vi "RichToFlatrouteguide_Rectangle.vi"(5 "OutputClusterType":T1, 11 "InputCluster":T3) -> (3 "OutputCluster":T1)   [LabVIEW 2019, in "Generated_server.lvlib"]
uses:
  Generated_server.lvlib
  routeguide_Rectangle.ctl
  routeguide_Point.ctl
  routeguide_Rectangle_Flat.ctl
  routeguide_Point_Flat.ctl
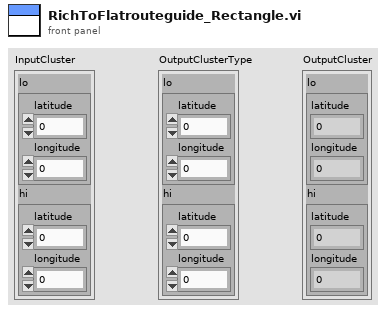
[diagram p1: front panel]
types:
  T1 = typedef "Generated_server.lvlib/routeguide_Rectangle_Flat.ctl" = cluster{"lo":T2, "hi":T2}
  T2 = typedef "Generated_server.lvlib/routeguide_Point_Flat.ctl" = cluster{"latitude":i32, "longitude":i32}
  T3 = typedef "Generated_server.lvlib/routeguide_Rectangle.ctl" = cluster{"lo":T4, "hi":T4}
  T4 = typedef "Generated_server.lvlib/routeguide_Point.ctl" = cluster{"latitude":i32, "longitude":i32}
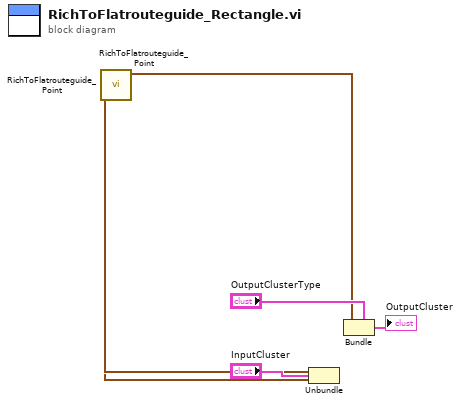
[diagram p0: block diagram]
diagram:
  n1 = Unbundle "Unbundle"("InputCluster") -> ("lo"=w4:T4, "hi"=w2:T4)
  n2 = call "RichToFlatrouteguide_Point.vi"("InputCluster"=w2) -> ("OutputCluster"=w1:T2)  [unwired: 10 in]
  n3 = call "RichToFlatrouteguide_Point.vi"("InputCluster"=w4) -> ("OutputCluster"=w3:T2)  [unwired: 10 in]
  n4 = Bundle "Bundle"(cluster="OutputClusterType", "lo"=w3, "hi"=w1) -> (→"OutputCluster":T1)
